vi "led_array.vi"(4 "error in":errorcluster, 7 "LED configuration":string="{\n\t\"actor_id\": \"\",\n\t\"attach_socket\": \"\",\n\t\"description\": \"\",\n\t\"enable_streaming\": true,\n\t\"lights\": [{\n\t\t\"array_id\": \"LF\",\n\t\t\"attach_socket\": \"\",\n\t\t\"coneLights\": [{\n\t\t\t\"attach_socket\": \"\",\n\t\t\t\"attenuation_radius\": 5000.0,\n\t\t\t\"backlight_attenuation_radius\": 20.0,\n\t\t\t\"backlight_color\": {\n\t\t\t\t\"a\": 255,\n\t\t\t\t\"b\": 255,\n\t\t\t\t\"g\": 255,\n\t\t\t\t\"r\": 255\n\t\t\t},\n\t\t\t\"backlight_indirect_lighting_intensity\": 10.0,\n\t\t\t\"backlight_intensity\": 400.0,\n\t\t\t\"backlight_location\": {\n\t\t\t\t\"x\": 0.0,\n\t\t\t\t\"y\": 0.0,\n\t\t\t\t\"z\": 0.0\n\t\t\t},\n\t\t\t\"backlight_soft_source_radius\": 2.0,\n\t\t\t\"backlight_source_length\": 1.0,\n\t\t\t\"backlight_source_radius\": 1.0,\n\t\t\t\"backlight_temperature\": 8000.0,\n\t\t\t\"backlight_volumetric_scattering_intensity\": 10.0,\n\t\t\t\"color\": {\n\t\t\t\t\"a\": 255,\n\t\t\t\t\"b\": 255,\n\t\t\t\t\"g\": 255,\n\t\t\t\t\"r\": 255\n\t\t\t},\n\t\t\t\"description\": \"\",\n\t\t\t\"enable_backlight\": true,\n\t\t\t\"enable_directional_light\": true,\n\t\t\t\"enable_streaming\": true,\n\t\t\t\"ies_profile\": \"\",\n\t\t\t\"indirect_lighting_intensity\": 1.0,\n\t\t\t\"inner_cone_angle\": 2.0,\n\t\t\t\"intensity\": 1500.0,\n\t\t\t\"led\": 0,\n\t\t\t\"listen_port\": 0,\n\t\t\t\"location\": {\n\t\t\t\t\"x\": 0.0,\n\t\t\t\t\"y\": 0.0,\n\t\t\t\t\"z\": 0.0\n\t\t\t},\n\t\t\t\"outer_cone_angle\": 6.0,\n\t\t\t\"parent_component_attachment\": \"\",\n\t\t\t\"raytrace_global_ilum\": false,\n\t\t\t\"raytrace_reflection\": false,\n\t\t\t\"raytrace_shadow\": false,\n\t\t\t\"receive_stream\": true,\n\t\t\t\"rotation\": {\n\t\t\t\t\"pitch\": -1.0,\n\t\t\t\t\"roll\": 0.0,\n\t\t\t\t\"yaw\": 6.0\n\t\t\t},\n\t\t\t\"soft_source_radius\": 0.0,\n\t\t\t\"source_length\": 1.0,\n\t\t\t\"source_radius\": 0.0,\n\t\t\t\"temperature\": 8000.0,\n\t\t\t\"type\": \"None\",\n\t\t\t\"use_attach_socket\": false,\n\t\t\t\"use_parent_component_attachment\": false,\n\t\t\t\"volumetric_scattering_intensity\": 5.0,\n\t\t\t\"wait_for_fresh_frame\": true\n\t\t}, {\n\t\t\t\"attach_socket\": \"\",\n\t\t\t\"attenuation_radius\": 5000.0,\n\t\t\t\"backlight_attenuation_radius\": 20.0,\n\t\t\t\"backlight_color\": {\n\t\t\t\t\"a\": 255,\n\t\t\t\t\"b\": 255,\n\t\t\t\t\"g\": 255,\n\t\t\t\t\"r\": 255\n\t\t\t},\n\t\t\t\"backlight_indirect_lighting_intensity\": 10.0,\n\t\t\t\"backlight_intensity\": 400.0,\n\t\t\t\"backlight_location\": {\n\t\t\t\t\"x\": 0.0,\n\t\t\t\t\"y\": 0.0,\n\t\t\t\t\"z\": 0.0\n\t\t\t},\n\t\t\t\"backlight_soft_source_radius\": 2.0,\n\t\t\t\"backlight_source_length\": 1.0,\n\t\t\t\"backlight_source_radius\": 1.0,\n\t\t\t\"backlight_temperature\": 8000.0,\n\t\t\t\"backlight_volumetric_scattering_intensity\": 10.0,\n\t\t\t\"color\": {\n\t\t\t\t\"a\": 255,\n\t\t\t\t\"b\": 255,\n\t\t\t\t\"g\": 255,\n\t\t\t\t\"r\": 255\n\t\t\t},\n\t\t\t\"description\": \"\",\n\t\t\t\"enable_backlight\": true,\n\t\t\t\"enable_directional_light\": true,\n\t\t\t\"enable_streaming\": true,\n\t\t\t\"ies_profile\": \"\",\n\t\t\t\"indirect_lighting_intensity\": 1.0,\n\t\t\t\"inner_cone_angle\": 2.0,\n\t\t\t\"intensity\": 1500.0,\n\t\t\t\"led\": 1,\n\t\t\t\"listen_port\": 0,\n\t\t\t\"location\": {\n\t\t\t\t\"x\": 0.0,\n\t\t\t\t\"y\": -2.0,\n\t\t\t\t\"z\": 0.0\n\t\t\t},\n\t\t\t\"outer_cone_angle\": 6.0,\n\t\t\t\"parent_component_attachment\": \"\",\n\t\t\t\"raytrace_global_ilum\": false,\n\t\t\t\"raytrace_reflection\": false,\n\t\t\t\"raytrace_shadow\": false,\n\t\t\t\"receive_stream\": true,\n\t\t\t\"rotation\": {\n\t\t\t\t\"pitch\": -1.0,\n\t\t\t\t\"roll\": 0.0,\n\t\t\t\t\"yaw\": 3.0\n\t\t\t},\n\t\t\t\"soft_source_radius\": 0.0,\n\t\t\t\"source_length\": 1.0,\n\t\t\t\"source_radius\": 0.0,\n\t\t\t\"temperature\": 8000.0,\n\t\t\t\"type\": \"None\",\n\t\t\t\"use_attach_socket\": false,\n\t\t\t\"use_parent_component_attachment\": false,\n\t\t\t\"volumetric_scattering_intensity\": 5.0,\n\t\t\t\"wait_for_fresh_frame\": true\n\t\t}, {\n\t\t\t\"attach_socket\": \"\",\n\t\t\t\"attenuation_radius\": 5000.0,\n\t\t\t\"backlight_attenuation_radius\": 20.0,\n\t\t\t\"backlight_color\": {\n\t\t\t\t\"a\": 255,\n\t\t\t\t\"b\": 255,\n\t\t\t\t\"g\": 255,\n\t\t\t\t\"r\": 255\n\t\t\t},\n\t\t\t\"backlight_indirect_lighting_intensity\": 10.0,\n\t\t\t\"backlight_intensity\": 400.0,\n\t\t\t\"backlight_location\": {\n\t\t\t\t\"x\": 0.0,\n\t\t\t\t\"y\": 0.0,\n\t\t\t\t\"z\": 0.0\n\t\t\t},\n\t\t\t\"backlight_soft_source_radius\": 2.0,\n\t\t\t\"backlight_source_length\": 1.0,\n\t\t\t\"backlight_source_radius\": 1.0,\n\t\t\t\"backlight_temperature\": 8000.0,\n\t\t\t\"backlight_volumetric_scattering_intensity\": 10.0,\n\t\t\t\"color\": {\n\t\t\t\t\"a\": 255,\n\t\t\t\t\"b\": 255,\n\t\t\t\t\"g\": 255,\n\t\t\t\t\"r\": 255\n\t\t\t},\n\t\t\t\"description\": \"\",\n\t\t\t\"enable_backlight\": true,\n\t\t\t\"enable_directional_light\": true,\n\t\t\t\"enable_streaming\": true,\n\t\t\t\"ies_profile\": \"\",\n\t\t\t\"indirect_lighting_intensity\": 1.0,\n\t\t\t\"inner_cone_angle\": 2.0,\n\t\t\t\"intensity\": 1500.0,\n\t\t\t\"led\": 2,\n\t\t\t\"listen_port\": 0,\n\t\t\t\"location\": {\n\t\t\t\t\"x\": 0.0,\n\t\t\t\t\"y\": -4.0,\n\t\t\t\t\"z\": 0.0\n\t\t\t},\n\t\t\t\"outer_cone_angle\": 6.0,\n\t\t\t\"parent_component_attachment\": \"\",\n\t\t\t\"raytrace_global_ilum\": false,\n\t\t\t\"raytrace_reflection\": false,\n\t\t\t\"raytrace_shadow\": false,\n\t\t\t\"receive_stream\": true,\n\t\t\t\"rotation\": {\n\t\t\t\t\"pitch\": -1.0,\n\t\t\t\t\"roll\": 0.0,\n\t\t\t\t\"yaw\": 0.0\n\t\t\t},\n\t\t\t\"soft_source_radius\": 0.0,\n\t\t\t\"source_length\": 1.0,\n\t\t\t\"source_radius\": 0.0,\n\t\t\t\"temperature\": 8000.0,\n\t\t\t\"type\": \"None\",\n\t\t\t\"use_attach_socket\": false,\n\t\t\t\"use_parent_component_attachment\": false,\n\t\t\t\"volumetric_scattering_intensity\": 5.0,\n\t\t\t\"wait_for_fresh_frame\": true\n\t\t}, {\n\t\t\t\"attach_socket\": \"\",\n\t\t\t\"attenuation_radius\": 5000.0,\n\t\t\t\"backlight_attenuation_radius\": 20.0,\n\t\t\t\"backlight_color\": {\n\t\t\t\t\"a\": 255,\n\t\t\t\t\"b\": 255,\n\t\t\t\t\"g\": 255,\n\t\t\t\t\"r\": 255\n\t\t\t},\n\t\t\t\"backlight_indirect_lighting_intensity\": 10.0,\n\t\t\t\"backlight_intensity\": 400.0,\n\t\t\t\"backlight_location\": {\n\t\t\t\t\"x\": 0.0,\n\t\t\t\t\"y\": 0.0,\n\t\t\t\t\"z\": 0.0\n\t\t\t},\n\t\t\t\"backlight_soft_source_radius\": 2.0,\n\t\t\t\"backlight_source_length\": 1.0,\n\t\t\t\"backlight_source_radius\": 1.0,\n\t\t\t\"backlight_temperature\": 8000.0,\n\t\t\t\"backlight_volumetric_scattering_intensity\": 10.0,\n\t\t\t\"color\": {\n\t\t\t\t\"a\": 255,\n\t\t\t\t\"b\": 255,\n\t\t\t\t\"g\": 255,\n\t\t\t\t\"r\": 255\n\t\t\t},\n\t\t\t\"description\": \"\",\n\t\t\t\"enable_backlight\": true,\n\t\t\t\"enable_directional_light\": true,\n\t\t\t\"enable_streaming\": true,\n\t\t\t\"ies_profile\": \"\",\n\t\t\t\"indirect_lighting_intensity\": 1.0,\n\t\t\t\"inner_cone_angle\": 2.0,\n\t\t\t\"intensity\": 1500.0,\n\t\t\t\"led\": 3,\n\t\t\t\"listen_port\": 0,\n\t\t\t\"location\": {\n\t\t\t\t\"x\": 0.0,\n\t\t\t\t\"y\": -6.0,\n\t\t\t\t\"z\": 0.0\n\t\t\t},\n\t\t\t\"outer_cone_angle\": 6.0,\n\t\t\t\"parent_component_attachment\": \"\",\n\t\t\t\"raytrace_global_ilum\": false,\n\t\t\t\"raytrace_reflection\": false,\n\t\t\t\"raytrace_shadow\": false,\n\t\t\t\"receive_stream\": true,\n\t\t\t\"rotation\": {\n\t\t\t\t\"pitch\": -1.0,\n\t\t\t\t\"roll\": 0.0,\n\t\t\t\t\"yaw\": -3.0\n\t\t\t},\n\t\t\t\"soft_source_radius\": 0.0,\n\t\t\t\"source_length\": 1.0,\n\t\t\t\"source_radius\": 0.0,\n\t\t\t\"temperature\": 8000.0,\n\t\t\t\"type\": \"None\",\n\t\t\t\"use_attach_socket\": false,\n\t\t\t\"use_parent_component_attachment\": false,\n\t\t\t\"volumetric_scattering_intensity\": 5.0,\n\t\t\t\"wait_for_fresh_frame\": true\n\t\t}, {\n\t\t\t\"attach_socket\": \"\",\n\t\t\t\"attenuation_radius\": 5000.0,\n\t\t\t\"backlight_attenuation_radius\": 20.0,\n\t\t\t\"backlight_color\": {\n\t\t\t\t\"a\": 255,\n\t\t\t\t\"b\": 255,\n\t\t\t\t\"g\": 255,\n\t\t\t\t\"r\": 255\n\t\t\t},\n\t\t\t\"backlight_indirect_lighting_intensity\": 10.0,\n\t\t\t\"backlight_intensity\": 400.0,\n\t\t\t\"backlight_location\": {\n\t\t\t\t\"x\": 0.0,\n\t\t\t\t\"y\": 0.0,\n\t\t\t\t\"z\": 0.0\n\t\t\t},\n\t\t\t\"backlight_soft_source_radius\": 2.0,\n\t\t\t\"backlight_source_length\": 1.0,\n\t\t\t\"backlight_source_radius\": 1.0,\n\t\t\t\"backlight_temperature\": 8000.0,\n\t\t\t\"backlight_volumetric_scattering_intensity\": 10.0,\n\t\t\t\"color\": {\n\t\t\t\t\"a\": 255,\n\t\t\t\t\"b\": 255,\n\t\t\t\t\"g\": 255,\n\t\t\t\t\"r\": 255\n\t\t\t},\n\t\t\t\"description\": \"\",\n\t\t\t\"enable_backlight\": true,\n\t\t\t\"enable_directional_light\": true,\n\t\t\t\"enable_streaming\": true,\n\t\t\t\"ies_profile\": \"\",\n\t\t\t\"indirect_lighting_intensity\": 1.0,\n\t\t\t\"inner_cone_angle\": 2.0,\n\t\t\t\"intensity\": 1500.0,\n\t\t\t\"led\": 4,\n\t\t\t\"listen_port\": 0,\n\t\t\t\"location\": {\n\t\t\t\t\"x\": 0.0,\n\t\t\t\t\"y\": -8.0,\n\t\t\t\t\"z\": 0.0\n\t\t\t},\n\t\t\t\"outer_cone_angle\": 6.0,\n\t\t\t\"parent_component_attachment\": \"\",\n\t\t\t\"raytrace_global_ilum\": false,\n\t\t\t\"raytrace_reflection\": false,\n\t\t\t\"raytrace_shadow\": false,\n\t\t\t\"receive_stream\": true,\n\t\t\t\"rotation\": {\n\t\t\t\t\"pitch\": -1.0,\n\t\t\t\t\"roll\": 0.0,\n\t\t\t\t\"yaw\": -6.0\n\t\t\t},\n\t\t\t\"soft_source_radius\": 0.0,\n\t\t\t\"source_length\": 1.0,\n\t\t\t\"source_radius\": 0.0,\n\t\t\t\"temperature\": 8000.0,\n\t\t\t\"type\": \"None\",\n\t\t\t\"use_attach_socket\": false,\n\t\t\t\"use_parent_component_attachment\": false,\n\t\t\t\"volumetric_scattering_intensity\": 5.0,\n\t\t\t\"wait_for_fresh_frame\": true\n\t\t}, {\n\t\t\t\"attach_socket\": \"\",\n\t\t\t\"attenuation_radius\": 5000.0,\n\t\t\t\"backlight_attenuation_radius\": 20.0,\n\t\t\t\"backlight_color\": {\n\t\t\t\t\"a\": 255,\n\t\t\t\t\"b\": 255,\n\t\t\t\t\"g\": 255,\n\t\t\t\t\"r\": 255\n\t\t\t},\n\t\t\t\"backlight_indirect_lighting_intensity\": 10.0,\n\t\t\t\"backlight_intensity\": 400.0,\n\t\t\t\"backlight_location\": {\n\t\t\t\t\"x\": 0.0,\n\t\t\t\t\"y\": 0.0,\n\t\t\t\t\"z\": 0.0\n\t\t\t},\n\t\t\t\"backlight_soft_source_radius\": 2.0,\n\t\t\t\"backlight_source_length\": 1.0,\n\t\t\t\"backlight_source_radius\": 1.0,\n\t\t\t\"backlight_temperature\": 8000.0,\n\t\t\t\"backlight_volumetric_scattering_intensity\": 10.0,\n\t\t\t\"color\": {\n\t\t\t\t\"a\": 255,\n\t\t\t\t\"b\": 255,\n\t\t\t\t\"g\": 255,\n\t\t\t\t\"r\": 255\n\t\t\t},\n\t\t\t\"description\": \"\",\n\t\t\t\"enable_backlight\": true,\n\t\t\t\"enable_directional_light\": true,\n\t\t\t\"enable_streaming\": true,\n\t\t\t\"ies_profile\": \"\",\n\t\t\t\"indirect_lighting_intensity\": 1.0,\n\t\t\t\"inner_cone_angle\": 2.0,\n\t\t\t\"intensity\": 1500.0,\n\t\t\t\"led\": 5,\n\t\t\t\"listen_port\": 0,\n\t\t\t\"location\": {\n\t\t\t\t\"x\": 0.0,\n\t\t\t\t\"y\": -10.0,\n\t\t\t\t\"z\": 0.0\n\t\t\t},\n\t\t\t\"outer_cone_angle\": 6.0,\n\t\t\t\"parent_component_attachment\": \"\",\n\t\t\t\"raytrace_global_ilum\": false,\n\t\t\t\"raytrace_reflection\": false,\n\t\t\t\"raytrace_shadow\": false,\n\t\t\t\"receive_stream\": true,\n\t\t\t\"rotation\": {\n\t\t\t\t\"pitch\": -1.0,\n\t\t\t\t\"roll\": 0.0,\n\t\t\t\t\"yaw\": -9.0\n\t\t\t},\n\t\t\t\"soft_source_radius\": 0.0,\n\t\t\t\"source_length\": 1.0,\n\t\t\t\"source_radius\": 0.0,\n\t\t\t\"temperature\": 8000.0,\n\t\t\t\"type\": \"None\",\n\t\t\t\"use_attach_socket\": false,\n\t\t\t\"use_parent_component_attachment\": false,\n\t\t\t\"volumetric_scattering_intensity\": 5.0,\n\t\t\t\"wait_for_fresh_frame\": true\n\t\t}, {\n\t\t\t\"attach_socket\": \"\",\n\t\t\t\"attenuation_radius\": 5000.0,\n\t\t\t\"backlight_attenuation_radius\": 20.0,\n\t\t\t\"backlight_color\": {\n\t\t\t\t\"a\": 255,\n\t\t\t\t\"b\": 255,\n\t\t\t\t\"g\": 255,\n\t\t\t\t\"r\": 255\n\t\t\t},\n\t\t\t\"backlight_indirect_lighting_intensity\": 10.0,\n\t\t\t\"backlight_intensity\": 400.0,\n\t\t\t\"backlight_location\": {\n\t\t\t\t\"x\": 0.0,\n\t\t\t\t\"y\": 0.0,\n\t\t\t\t\"z\": 0.0\n\t\t\t},\n\t\t\t\"backlight_soft_source_radius\": 2.0,\n\t\t\t\"backlight_source_length\": 1.0,\n\t\t\t\"backlight_source_radius\": 1.0,\n\t\t\t\"backlight_temperature\": 8000.0,\n\t\t\t\"backlight_volumetric_scattering_intensity\": 10.0,\n\t\t\t\"color\": {\n\t\t\t\t\"a\": 255,\n\t\t\t\t\"b\": 255,\n\t\t\t\t\"g\": 255,\n\t\t\t\t\"r\": 255\n\t\t\t},\n\t\t\t\"description\": \"\",\n\t\t\t\"enable_backlight\": true,\n\t\t\t\"enable_directional_light\": true,\n\t\t\t\"enable_streaming\": true,\n\t\t\t\"ies_profile\": \"\",\n\t\t\t\"indirect_lighting_intensity\": 1.0,\n\t\t\t\"inner_cone_angle\": 2.0,\n\t\t\t\"intensity\": 1500.0,\n\t\t\t\"led\": 6,\n\t\t\t\"listen_port\": 0,\n\t\t\t\"location\": {\n\t\t\t\t\"x\": 0.0,\n\t\t\t\t\"y\": -12.0,\n\t\t\t\t\"z\": 0.0\n\t\t\t},\n\t\t\t\"outer_cone_angle\": 6.0,\n\t\t\t\"parent_component_attachment\": \"\",\n\t\t\t\"raytrace_global_ilum\": false,\n\t\t\t\"raytrace_reflection\": false,\n\t\t\t\"raytrace_shadow\": false,\n\t\t\t\"receive_stream\": true,\n\t\t\t\"rotation\": {\n\t\t\t\t\"pitch\": -1.0,\n\t\t\t\t\"roll\": 0.0,\n\t\t\t\t\"yaw\": -12.0\n\t\t\t},\n\t\t\t\"soft_source_radius\": 0.0,\n\t\t\t\"source_length\": 1.0,\n\t\t\t\"source_radius\": 0.0,\n\t\t\t\"temperature\": 8000.0,\n\t\t\t\"type\": \"None\",\n\t\t\t\"use_attach_socket\": false,\n\t\t\t\"use_parent_component_attachment\": false,\n\t\t\t\"volumetric_scattering_intensity\": 5.0,\n\t\t\t\"wait_for_fresh_frame\": true\n\t\t}, {\n\t\t\t\"attach_socket\": \"\",\n\t\t\t\"attenuation_radius\": 5000.0,\n\t\t\t\"backlight_attenuation_radius\": 20.0,\n\t\t\t\"backlight_color\": {\n\t\t\t\t\"a\": 255,\n\t\t\t\t\"b\": 255,\n\t\t\t\t\"g\": 255,\n\t\t\t\t\"r\": 255\n\t\t\t},\n\t\t\t\"backlight_indirect_lighting_intensity\": 10.0,\n\t\t\t\"backlight_intensity\": 400.0,\n\t\t\t\"backlight_location\": {\n\t\t\t\t\"x\": 0.0,\n\t\t\t\t\"y\": 0.0,\n\t\t\t\t\"z\": 0.0\n\t\t\t},\n\t\t\t\"backlight_soft_source_radius\": 2.0,\n\t\t\t\"backlight_source_length\": 1.0,\n\t\t\t\"backlight_source_radius\": 1.0,\n\t\t\t\"backlight_temperature\": 8000.0,\n\t\t\t\"backlight_volumetric_scattering_intensity\": 10.0,\n\t\t\t\"color\": {\n\t\t\t\t\"a\": 255,\n\t\t\t\t\"b\": 255,\n\t\t\t\t\"g\": 255,\n\t\t\t\t\"r\": 255\n\t\t\t},\n\t\t\t\"description\": \"\",\n\t\t\t\"enable_backlight\": true,\n\t\t\t\"enable_directional_light\": true,\n\t\t\t\"enable_streaming\": true,\n\t\t\t\"ies_profile\": \"\",\n\t\t\t\"indirect_lighting_intensity\": 1.0,\n\t\t\t\"inner_cone_angle\": 2.0,\n\t\t\t\"intensity\": 1500.0,\n\t\t\t\"led\": 7,\n\t\t\t\"listen_port\": 0,\n\t\t\t\"location\": {\n\t\t\t\t\"x\": 0.0,\n\t\t\t\t\"y\": -14.0,\n\t\t\t\t\"z\": 0.0\n\t\t\t},\n\t\t\t\"outer_cone_angle\": 6.0,\n\t\t\t\"parent_component_attachment\": \"\",\n\t\t\t\"raytrace_global_ilum\": false,\n\t\t\t\"raytrace_reflection\": false,\n\t\t\t\"raytrace_shadow\": false,\n\t\t\t\"receive_stream\": true,\n\t\t\t\"rotation\": {\n\t\t\t\t\"pitch\": -1.0,\n\t\t\t\t\"roll\": 0.0,\n\t\t\t\t\"yaw\": -15.0\n\t\t\t},\n\t\t\t\"soft_source_radius\": 0.0,\n\t\t\t\"source_length\": 1.0,\n\t\t\t\"source_radius\": 0.0,\n\t\t\t\"temperature\": 8000.0,\n\t\t\t\"type\": \"None\",\n\t\t\t\"use_attach_socket\": false,\n\t\t\t\"use_parent_component_attachment\": false,\n\t\t\t\"volumetric_scattering_intensity\": 5.0,\n\t\t\t\"wait_for_fresh_frame\": true\n\t\t}],\n\t\t\"description\": \"\",\n\t\t\"enable_streaming\": true,\n\t\t\"listen_port\": 0,\n\t\t\"location\": {\n\t\t\t\"x\": 200.57719399999999155,\n\t\t\t\"y\": -79.397000000000005571,\n\t\t\t\"z\": 83.918998999999999455\n\t\t},\n\t\t\"parent_component_attachment\": \"\",\n\t\t\"receive_stream\": true,\n\t\t\"rectLights\": [],\n\t\t\"rotation\": {\n\t\t\t\"pitch\": 0.0,\n\t\t\t\"roll\": 0.0,\n\t\t\t\"yaw\": 0.0\n\t\t},\n\t\t\"type\": \"None\",\n\t\t\"use_attach_socket\": false,\n\t\t\"use_parent_component_attachment\": false,\n\t\t\"wait_for_fresh_frame\": true\n\t}, {\n\t\t\"array_id\": \"RF\",\n\t\t\"attach_socket\": \"\",\n\t\t\"coneLights\": [{\n\t\t\t\"attach_socket\": \"\",\n\t\t\t\"attenuation_radius\": 5000.0,\n\t\t\t\"backlight_attenuation_radius\": 20.0,\n\t\t\t\"backlight_color\": {\n\t\t\t\t\"a\": 255,\n\t\t\t\t\"b\": 255,\n\t\t\t\t\"g\": 255,\n\t\t\t\t\"r\": 255\n\t\t\t},\n\t\t\t\"backlight_indirect_lighting_intensity\": 10.0,\n\t\t\t\"backlight_intensity\": 400.0,\n\t\t\t\"backlight_location\": {\n\t\t\t\t\"x\": 0.0,\n\t\t\t\t\"y\": 0.0,\n\t\t\t\t\"z\": 0.0\n\t\t\t},\n\t\t\t\"backlight_soft_source_radius\": 2.0,\n\t\t\t\"backlight_source_length\": 1.0,\n\t\t\t\"backlight_source_radius\": 1.0,\n\t\t\t\"backlight_temperature\": 8000.0,\n\t\t\t\"backlight_volumetric_scattering_intensity\": 10.0,\n\t\t\t\"color\": {\n\t\t\t\t\"a\": 255,\n\t\t\t\t\"b\": 255,\n\t\t\t\t\"g\": 255,\n\t\t\t\t\"r\": 255\n\t\t\t},\n\t\t\t\"description\": \"\",\n\t\t\t\"enable_backlight\": true,\n\t\t\t\"enable_directional_light\": true,\n\t\t\t\"enable_streaming\": true,\n\t\t\t\"ies_profile\": \"\",\n\t\t\t\"indirect_lighting_intensity\": 1.0,\n\t\t\t\"inner_cone_angle\": 2.0,\n\t\t\t\"intensity\": 1500.0,\n\t\t\t\"led\": 0,\n\t\t\t\"listen_port\": 0,\n\t\t\t\"location\": {\n\t\t\t\t\"x\": 0.0,\n\t\t\t\t\"y\": 0.0,\n\t\t\t\t\"z\": 0.0\n\t\t\t},\n\t\t\t\"outer_cone_angle\": 6.0,\n\t\t\t\"parent_component_attachment\": \"\",\n\t\t\t\"raytrace_global_ilum\": false,\n\t\t\t\"raytrace_reflection\": false,\n\t\t\t\"raytrace_shadow\": false,\n\t\t\t\"receive_stream\": true,\n\t\t\t\"rotation\": {\n\t\t\t\t\"pitch\": -1.0,\n\t\t\t\t\"roll\": 0.0,\n\t\t\t\t\"yaw\": -6.0\n\t\t\t},\n\t\t\t\"soft_source_radius\": 0.0,\n\t\t\t\"source_length\": 1.0,\n\t\t\t\"source_radius\": 0.0,\n\t\t\t\"temperature\": 8000.0,\n\t\t\t\"type\": \"None\",\n\t\t\t\"use_attach_socket\": false,\n\t\t\t\"use_parent_component_attachment\": false,\n\t\t\t\"volumetric_scattering_intensity\": 5.0,\n\t\t\t\"wait_for_fresh_frame\": true\n\t\t}, {\n\t\t\t\"attach_socket\": \"\",\n\t\t\t\"attenuation_radius\": 5000.0,\n\t\t\t\"backlight_attenuation_radius\": 20.0,\n\t\t\t\"backlight_color\": {\n\t\t\t\t\"a\": 255,\n\t\t\t\t\"b\": 255,\n\t\t\t\t\"g\": 255,\n\t\t\t\t\"r\": 255\n\t\t\t},\n\t\t\t\"backlight_indirect_lighting_intensity\": 10.0,\n\t\t\t\"backlight_intensity\": 400.0,\n\t\t\t\"backlight_location\": {\n\t\t\t\t\"x\": 0.0,\n\t\t\t\t\"y\": 0.0,\n\t\t\t\t\"z\": 0.0\n\t\t\t},\n\t\t\t\"backlight_soft_source_radius\": 2.0,\n\t\t\t\"backlight_source_length\": 1.0,\n\t\t\t\"backlight_source_radius\": 1.0,\n\t\t\t\"backlight_temperature\": 8000.0,\n\t\t\t\"backlight_volumetric_scattering_intensity\": 10.0,\n\t\t\t\"color\": {\n\t\t\t\t\"a\": 255,\n\t\t\t\t\"b\": 255,\n\t\t\t\t\"g\": 255,\n\t\t\t\t\"r\": 255\n\t\t\t},\n\t\t\t\"description\": \"\",\n\t\t\t\"enable_backlight\": true,\n\t\t\t\"enable_directional_light\": true,\n\t\t\t\"enable_streaming\": true,\n\t\t\t\"ies_profile\": \"\",\n\t\t\t\"indirect_lighting_intensity\": 1.0,\n\t\t\t\"inner_cone_angle\": 2.0,\n\t\t\t\"intensity\": 1500.0,\n\t\t\t\"led\": 1,\n\t\t\t\"listen_port\": 0,\n\t\t\t\"location\": {\n\t\t\t\t\"x\": 0.0,\n\t\t\t\t\"y\": 2.0,\n\t\t\t\t\"z\": 0.0\n\t\t\t},\n\t\t\t\"outer_cone_angle\": 6.0,\n\t\t\t\"parent_component_attachment\": \"\",\n\t\t\t\"raytrace_global_ilum\": false,\n\t\t\t\"raytrace_reflection\": false,\n\t\t\t\"raytrace_shadow\": false,\n\t\t\t\"receive_stream\": true,\n\t\t\t\"rotation\": {\n\t\t\t\t\"pitch\": -1.0,\n\t\t\t\t\"roll\": 0.0,\n\t\t\t\t\"yaw\": -3.0\n\t\t\t},\n\t\t\t\"soft_source_radius\": 0.0,\n\t\t\t\"source_length\": 1.0,\n\t\t\t\"source_radius\": 0.0,\n\t\t\t\"temperature\": 8000.0,\n\t\t\t\"type\": \"None\",\n\t\t\t\"use_attach_socket\": false,\n\t\t\t\"use_parent_component_attachment\": false,\n\t\t\t\"volumetric_scattering_intensity\": 5.0,\n\t\t\t\"wait_for_fresh_frame\": true\n\t\t}, {\n\t\t\t\"attach_socket\": \"\",\n\t\t\t\"attenuation_radius\": 5000.0,\n\t\t\t\"backlight_attenuation_radius\": 20.0,\n\t\t\t\"backlight_color\": {\n\t\t\t\t\"a\": 255,\n\t\t\t\t\"b\": 255,\n\t\t\t\t\"g\": 255,\n\t\t\t\t\"r\": 255\n\t\t\t},\n\t\t\t\"backlight_indirect_lighting_intensity\": 10.0,\n\t\t\t\"backlight_intensity\": 400.0,\n\t\t\t\"backlight_location\": {\n\t\t\t\t\"x\": 0.0,\n\t\t\t\t\"y\": 0.0,\n\t\t\t\t\"z\": 0.0\n\t\t\t},\n\t\t\t\"backlight_soft_source_radius\": 2.0,\n\t\t\t\"backlight_source_length\": 1.0,\n\t\t\t\"backlight_source_radius\": 1.0,\n\t\t\t\"backlight_temperature\": 8000.0,\n\t\t\t\"backlight_volumetric_scattering_intensity\": 10.0,\n\t\t\t\"color\": {\n\t\t\t\t\"a\": 255,\n\t\t\t\t\"b\": 255,\n\t\t\t\t\"g\": 255,\n\t\t\t\t\"r\": 255\n\t\t\t},\n\t\t\t\"description\": \"\",\n\t\t\t\"enable_backlight\": true,\n\t\t\t\"enable_directional_light\": true,\n\t\t\t\"enable_streaming\": true,\n\t\t\t\"ies_profile\": \"\",\n\t\t\t\"indirect_lighting_intensity\": 1.0,\n\t\t\t\"inner_cone_angle\": 2.0,\n\t\t\t\"intensity\": 1500.0,\n\t\t\t\"led\": 2,\n\t\t\t\"listen_port\": 0,\n\t\t\t\"location\": {\n\t\t\t\t\"x\": 0.0,\n\t\t\t\t\"y\": 4.0,\n\t\t\t\t\"z\": 0.0\n\t\t\t},\n\t\t\t\"outer_cone_angle\": 6.0,\n\t\t\t\"parent_component_attachment\": \"\",\n\t\t\t\"raytrace_global_ilum\": false,\n\t\t\t\"raytrace_reflection\": false,\n\t\t\t\"raytrace_shadow\": false,\n\t\t\t\"receive_stream\": true,\n\t\t\t\"rotation\": {\n\t\t\t\t\"pitch\": -1.0,\n\t\t\t\t\"roll\": 0.0,\n\t\t\t\t\"yaw\": 0.0\n\t\t\t},\n\t\t\t\"soft_source_radius\": 0.0,\n\t\t\t\"source_length\": 1.0,\n\t\t\t\"source_radius\": 0.0,\n\t\t\t\"temperature\": 8000.0,\n\t\t\t\"type\": \"None\",\n\t\t\t\"use_attach_socket\": false,\n\t\t\t\"use_parent_component_attachment\": false,\n\t\t\t\"volumetric_scattering_intensity\": 5.0,\n\t\t\t\"wait_for_fresh_frame\": true\n\t\t}, {\n\t\t\t\"attach_socket\": \"\",\n\t\t\t\"attenuation_radius\": 5000.0,\n\t\t\t\"backlight_attenuation_radius\": 20.0,\n\t\t\t\"backlight_color\": {\n\t\t\t\t\"a\": 255,\n\t\t\t\t\"b\": 255,\n\t\t\t\t\"g\": 255,\n\t\t\t\t\"r\": 255\n\t\t\t},\n\t\t\t\"backlight_indirect_lighting_intensity\": 10.0,\n\t\t\t\"backlight_intensity\": 400.0,\n\t\t\t\"backlight_location\": {\n\t\t\t\t\"x\": 0.0,\n\t\t\t\t\"y\": 0.0,\n\t\t\t\t\"z\": 0.0\n\t\t\t},\n\t\t\t\"backlight_soft_source_radius\": 2.0,\n\t\t\t\"backlight_source_length\": 1.0,\n\t\t\t\"backlight_source_radius\": 1.0,\n\t\t\t\"backlight_temperature\": 8000.0,\n\t\t\t\"backlight_volumetric_scattering_intensity\": 10.0,\n\t\t\t\"color\": {\n\t\t\t\t\"a\": 255,\n\t\t\t\t\"b\": 255,\n\t\t\t\t\"g\": 255,\n\t\t\t\t\"r\": 255\n\t\t\t},\n\t\t\t\"description\": \"\",\n\t\t\t\"enable_backlight\": true,\n\t\t\t\"enable_directional_light\": true,\n\t\t\t\"enable_streaming\": true,\n\t\t\t\"ies_profile\": \"\",\n\t\t\t\"indirect_lighting_intensity\": 1.0,\n\t\t\t\"inner_cone_angle\": 2.0,\n\t\t\t\"intensity\": 1500.0,\n\t\t\t\"led\": 3,\n\t\t\t\"listen_port\": 0,\n\t\t\t\"location\": {\n\t\t\t\t\"x\": 0.0,\n\t\t\t\t\"y\": 6.0,\n\t\t\t\t\"z\": 0.0\n\t\t\t},\n\t\t\t\"outer_cone_angle\": 6.0,\n\t\t\t\"parent_component_attachment\": \"\",\n\t\t\t\"raytrace_global_ilum\": false,\n\t\t\t\"raytrace_reflection\": false,\n\t\t\t\"raytrace_shadow\": false,\n\t\t\t\"receive_stream\": true,\n\t\t\t\"rotation\": {\n\t\t\t\t\"pitch\": -1.0,\n\t\t\t\t\"roll\": 0.0,\n\t\t\t\t\"yaw\": 3.0\n\t\t\t},\n\t\t\t\"soft_source_radius\": 0.0,\n\t\t\t\"source_length\": 1.0,\n\t\t\t\"source_radius\": 0.0,\n\t\t\t\"temperature\": 8000.0,\n\t\t\t\"type\": \"None\",\n\t\t\t\"use_attach_socket\": false,\n\t\t\t\"use_parent_component_attachment\": false,\n\t\t\t\"volumetric_scattering_intensity\": 5.0,\n\t\t\t\"wait_for_fresh_frame\": true\n\t\t}, {\n\t\t\t\"attach_socket\": \"\",\n\t\t\t\"attenuation_radius\": 5000.0,\n\t\t\t\"backlight_attenuation_radius\": 20.0,\n\t\t\t\"backlight_color\": {\n\t\t\t\t\"a\": 255,\n\t\t\t\t\"b\": 255,\n\t\t\t\t\"g\": 255,\n\t\t\t\t\"r\": 255\n\t\t\t},\n\t\t\t\"backlight_indirect_lighting_intensity\": 10.0,\n\t\t\t\"backlight_intensity\": 400.0,\n\t\t\t\"backlight_location\": {\n\t\t\t\t\"x\": 0.0,\n\t\t\t\t\"y\": 0.0,\n\t\t\t\t\"z\": 0.0\n\t\t\t},\n\t\t\t\"backlight_soft_source_radius\": 2.0,\n\t\t\t\"backlight_source_length\": 1.0,\n\t\t\t\"backlight_source_radius\": 1.0,\n\t\t\t\"backlight_temperature\": 8000.0,\n\t\t\t\"backlight_volumetric_scattering_intensity\": 10.0,\n\t\t\t\"color\": {\n\t\t\t\t\"a\": 255,\n\t\t\t\t\"b\": 255,\n\t\t\t\t\"g\": 255,\n\t\t\t\t\"r\": 255\n\t\t\t},\n\t\t\t\"description\": \"\",\n\t\t\t\"enable_backlight\": true,\n\t\t\t\"enable_directional_light\": true,\n\t\t\t\"enable_streaming\": true,\n\t\t\t\"ies_profile\": \"\",\n\t\t\t\"indirect_lighting_intensity\": 1.0,\n\t\t\t\"inner_cone_angle\": 2.0,\n\t\t\t\"intensity\": 1500.0,\n\t\t\t\"led\": 4,\n\t\t\t\"listen_port\": 0,\n\t\t\t\"location\": {\n\t\t\t\t\"x\": 0.0,\n\t\t\t\t\"y\": 8.0,\n\t\t\t\t\"z\": 0.0\n\t\t\t},\n\t\t\t\"outer_cone_angle\": 6.0,\n\t\t\t\"parent_component_attachment\": \"\",\n\t\t\t\"raytrace_global_ilum\": false,\n\t\t\t\"raytrace_reflection\": false,\n\t\t\t\"raytrace_shadow\": false,\n\t\t\t\"receive_stream\": true,\n\t\t\t\"rotation\": {\n\t\t\t\t\"pitch\": -1.0,\n\t\t\t\t\"roll\": 0.0,\n\t\t\t\t\"yaw\": 6.0\n\t\t\t},\n\t\t\t\"soft_source_radius\": 0.0,\n\t\t\t\"source_length\": 1.0,\n\t\t\t\"source_radius\": 0.0,\n\t\t\t\"temperature\": 8000.0,\n\t\t\t\"type\": \"None\",\n\t\t\t\"use_attach_socket\": false,\n\t\t\t\"use_parent_component_attachment\": false,\n\t\t\t\"volumetric_scattering_intensity\": 5.0,\n\t\t\t\"wait_for_fresh_frame\": true\n\t\t}, {\n\t\t\t\"attach_socket\": \"\",\n\t\t\t\"attenuation_radius\": 5000.0,\n\t\t\t\"backlight_attenuation_radius\": 20.0,\n\t\t\t\"backlight_color\": {\n\t\t\t\t\"a\": 255,\n\t\t\t\t\"b\": 255,\n\t\t\t\t\"g\": 255,\n\t\t\t\t\"r\": 255\n\t\t\t},\n\t\t\t\"backlight_indirect_lighting_intensity\": 10.0,\n\t\t\t\"backlight_intensity\": 400.0,\n\t\t\t\"backlight_location\": {\n\t\t\t\t\"x\": 0.0,\n\t\t\t\t\"y\": 0.0,\n\t\t\t\t\"z\": 0.0\n\t\t\t},\n\t\t\t\"backlight_soft_source_radius\": 2.0,\n\t\t\t\"backlight_source_length\": 1.0,\n\t\t\t\"backlight_source_radius\": 1.0,\n\t\t\t\"backlight_temperature\": 8000.0,\n\t\t\t\"backlight_volumetric_scattering_intensity\": 10.0,\n\t\t\t\"color\": {\n\t\t\t\t\"a\": 255,\n\t\t\t\t\"b\": 255,\n\t\t\t\t\"g\": 255,\n\t\t\t\t\"r\": 255\n\t\t\t},\n\t\t\t\"description\": \"\",\n\t\t\t\"enable_backlight\": true,\n\t\t\t\"enable_directional_light\": true,\n\t\t\t\"enable_streaming\": true,\n\t\t\t\"ies_profile\": \"\",\n\t\t\t\"indirect_lighting_intensity\": 1.0,\n\t\t\t\"inner_cone_angle\": 2.0,\n\t\t\t\"intensity\": 1500.0,\n\t\t\t\"led\": 5,\n\t\t\t\"listen_port\": 0,\n\t\t\t\"location\": {\n\t\t\t\t\"x\": 0.0,\n\t\t\t\t\"y\": 10.0,\n\t\t\t\t\"z\": 0.0\n\t\t\t},\n\t\t\t\"outer_cone_angle\": 6.0,\n\t\t\t\"parent_component_attachment\": \"\",\n\t\t\t\"raytrace_global_ilum\": false,\n\t\t\t\"raytrace_reflection\": false,\n\t\t\t\"raytrace_shadow\": false,\n\t\t\t\"receive_stream\": true,\n\t\t\t\"rotation\": {\n\t\t\t\t\"pitch\": -1.0,\n\t\t\t\t\"roll\": 0.0,\n\t\t\t\t\"yaw\": 9.0\n\t\t\t},\n\t\t\t\"soft_source_radius\": 0.0,\n\t\t\t\"source_length\": 1.0,\n\t\t\t\"source_radius\": 0.0,\n\t\t\t\"temperature\": 8000.0,\n\t\t\t\"type\": \"None\",\n\t\t\t\"use_attach_socket\": false,\n\t\t\t\"use_parent_component_attachment\": false,\n\t\t\t\"volumetric_scattering_intensity\": 5.0,\n\t\t\t\"wait_for_fresh_frame\": true\n\t\t}, {\n\t\t\t\"attach_socket\": \"\",\n\t\t\t\"attenuation_radius\": 5000.0,\n\t\t\t\"backlight_attenuation_radius\": 20.0,\n\t\t\t\"backlight_color\": {\n\t\t\t\t\"a\": 255,\n\t\t\t\t\"b\": 255,\n\t\t\t\t\"g\": 255,\n\t\t\t\t\"r\": 255\n\t\t\t},\n\t\t\t\"backlight_indirect_lighting_intensity\": 10.0,\n\t\t\t\"backlight_intensity\": 400.0,\n\t\t\t\"backlight_location\": {\n\t\t\t\t\"x\": 0.0,\n\t\t\t\t\"y\": 0.0,\n\t\t\t\t\"z\": 0.0\n\t\t\t},\n\t\t\t\"backlight_soft_source_radius\": 2.0,\n\t\t\t\"backlight_source_length\": 1.0,\n\t\t\t\"backlight_source_radius\": 1.0,\n\t\t\t\"backlight_temperature\": 8000.0,\n\t\t\t\"backlight_volumetric_scattering_intensity\": 10.0,\n\t\t\t\"color\": {\n\t\t\t\t\"a\": 255,\n\t\t\t\t\"b\": 255,\n\t\t\t\t\"g\": 255,\n\t\t\t\t\"r\": 255\n\t\t\t},\n\t\t\t\"description\": \"\",\n\t\t\t\"enable_backlight\": true,\n\t\t\t\"enable_directional_light\": true,\n\t\t\t\"enable_streaming\": true,\n\t\t\t\"ies_profile\": \"\",\n\t\t\t\"indirect_lighting_intensity\": 1.0,\n\t\t\t\"inner_cone_angle\": 2.0,\n\t\t\t\"intensity\": 1500.0,\n\t\t\t\"led\": 6,\n\t\t\t\"listen_port\": 0,\n\t\t\t\"location\": {\n\t\t\t\t\"x\": 0.0,\n\t\t\t\t\"y\": 12.0,\n\t\t\t\t\"z\": 0.0\n\t\t\t},\n\t\t\t\"outer_cone_angle\": 6.0,\n\t\t\t\"parent_component_attachment\": \"\",\n\t\t\t\"raytrace_global_ilum\": false,\n\t\t\t\"raytrace_reflection\": false,\n\t\t\t\"raytrace_shadow\": false,\n\t\t\t\"receive_stream\": true,\n\t\t\t\"rotation\": {\n\t\t\t\t\"pitch\": -1.0,\n\t\t\t\t\"roll\": 0.0,\n\t\t\t\t\"yaw\": 12.0\n\t\t\t},\n\t\t\t\"soft_source_radius\": 0.0,\n\t\t\t\"source_length\": 1.0,\n\t\t\t\"source_radius\": 0.0,\n\t\t\t\"temperature\": 8000.0,\n\t\t\t\"type\": \"None\",\n\t\t\t\"use_attach_socket\": false,\n\t\t\t\"use_parent_component_attachment\": false,\n\t\t\t\"volumetric_scattering_intensity\": 5.0,\n\t\t\t\"wait_for_fresh_frame\": true\n\t\t}, {\n\t\t\t\"attach_socket\": \"\",\n\t\t\t\"attenuation_radius\": 5000.0,\n\t\t\t\"backlight_attenuation_radius\": 20.0,\n\t\t\t\"backlight_color\": {\n\t\t\t\t\"a\": 255,\n\t\t\t\t\"b\": 255,\n\t\t\t\t\"g\": 255,\n\t\t\t\t\"r\": 255\n\t\t\t},\n\t\t\t\"backlight_indirect_lighting_intensity\": 10.0,\n\t\t\t\"backlight_intensity\": 400.0,\n\t\t\t\"backlight_location\": {\n\t\t\t\t\"x\": 0.0,\n\t\t\t\t\"y\": 0.0,\n\t\t\t\t\"z\": 0.0\n\t\t\t},\n\t\t\t\"backlight_soft_source_radius\": 2.0,\n\t\t\t\"backlight_source_length\": 1.0,\n\t\t\t\"backlight_source_radius\": 1.0,\n\t\t\t\"backlight_temperature\": 8000.0,\n\t\t\t\"backlight_volumetric_scattering_intensity\": 10.0,\n\t\t\t\"color\": {\n\t\t\t\t\"a\": 255,\n\t\t\t\t\"b\": 255,\n\t\t\t\t\"g\": 255,\n\t\t\t\t\"r\": 255\n\t\t\t},\n\t\t\t\"description\": \"\",\n\t\t\t\"enable_backlight\": true,\n\t\t\t\"enable_directional_light\": true,\n\t\t\t\"enable_streaming\": true,\n\t\t\t\"ies_profile\": \"\",\n\t\t\t\"indirect_lighting_intensity\": 1.0,\n\t\t\t\"inner_cone_angle\": 2.0,\n\t\t\t\"intensity\": 1500.0,\n\t\t\t\"led\": 7,\n\t\t\t\"listen_port\": 0,\n\t\t\t\"location\": {\n\t\t\t\t\"x\": 0.0,\n\t\t\t\t\"y\": 14.0,\n\t\t\t\t\"z\": 0.0\n\t\t\t},\n\t\t\t\"outer_cone_angle\": 6.0,\n\t\t\t\"parent_component_attachment\": \"\",\n\t\t\t\"raytrace_global_ilum\": false,\n\t\t\t\"raytrace_reflection\": false,\n\t\t\t\"raytrace_shadow\": false,\n\t\t\t\"receive_stream\": true,\n\t\t\t\"rotation\": {\n\t\t\t\t\"pitch\": -1.0,\n\t\t\t\t\"roll\": 0.0,\n\t\t\t\t\"yaw\": 15.0\n\t\t\t},\n\t\t\t\"soft_source_radius\": 0.0,\n\t\t\t\"source_length\": 1.0,\n\t\t\t\"source_radius\": 0.0,\n\t\t\t\"temperature\": 8000.0,\n\t\t\t\"type\": \"None\",\n\t\t\t\"use_attach_socket\": false,\n\t\t\t\"use_parent_component_attachment\": false,\n\t\t\t\"volumetric_scattering_intensity\": 5.0,\n\t\t\t\"wait_for_fresh_frame\": true\n\t\t}],\n\t\t\"description\": \"\",\n\t\t\"enable_streaming\": true,\n\t\t\"listen_port\": 0,\n\t\t\"location\": {\n\t\t\t\"x\": 200.57719399999999155,\n\t\t\t\"y\": 79.397000000000005571,\n\t\t\t\"z\": 83.918998999999999455\n\t\t},\n\t\t\"parent_component_attachment\": \"\",\n\t\t\"receive_stream\": true,\n\t\t\"rectLights\": [],\n\t\t\"rotation\": {\n\t\t\t\"pitch\": 0.0,\n\t\t\t\"roll\": 0.0,\n\t\t\t\"yaw\": 0.0\n\t\t},\n\t\t\"type\": \"None\",\n\t\t\"use_attach_socket\": false,\n\t\t\"use_parent_component_attachment\": false,\n\t\t\"wait_for_fresh_frame\": true\n\t}],\n\t\"listen_port\": 0,\n\t\"location\": {\n\t\t\"x\": 0.0,\n\t\t\"y\": 0.0,\n\t\t\"z\": 0.0\n\t},\n\t\"parent_component_attachment\": \"\",\n\t\"receive_stream\": true,\n\t\"rotation\": {\n\t\t\"pitch\": 0.0,\n\t\t\"roll\": 0.0,\n\t\t\"yaw\": 0.0\n\t},\n\t\"type\": \"None\",\n\t\"use_attach_socket\": false,\n\t\"use_parent_component_attachment\": false,\n\t\"wait_for_fresh_frame\": true\n}") -> (0 "error out":errorcluster)   [LabVIEW 2019]
doc: "Configures and updates an array of LEDs attached to the ego vehicle."
uses:
  controls/lights_state.ctl
  controls/lights_rect_cone.ctl
  tools/simx_common.vi
panel:
  out "Number of Lights Detected":i32=16
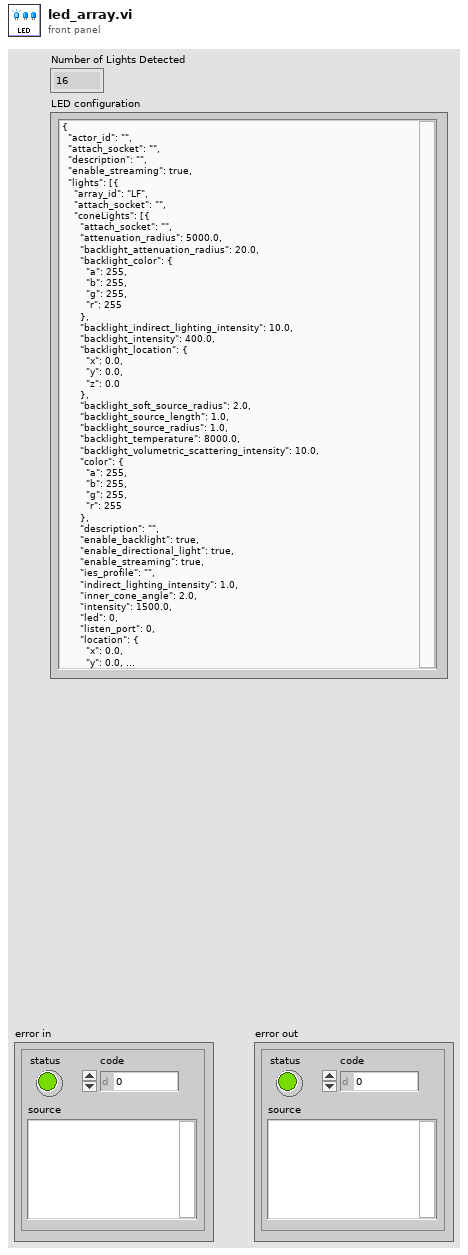
[diagram p1: front panel]
types:
  T1 = typedef "lights_state.ctl" = enum16{"Init", "Configure", "Update"}
  T2 = typedef "simx_connection.ctl" = cluster{"Config":T3, "Connections":T6, "Map":cluster{"lanes":cluster{"x":dbl[], "y":dbl[], "z":dbl[]}, "StartPosition":cluster{"start_points":T7, "StartRotation":dbl[], "StartLocation":dbl[]}, "Draw Map Size":T8, "DrawArea":cluster{"min_Y":dbl, "min_X":dbl, "Scale X":dbl, "Scale Y":dbl}, "Map":picture, "Map Geojson":string}}
  T3 = typedef "config.ctl" = cluster{"Trajectory":T4, "Weather":T5}
  T4 = typedef "trajectory.ctl" = cluster{"Number of frames":i32, "Frame number":i32, "Trajectory":string}
  T5 = typedef "weather.ctl" = cluster{"id":string}
  T6 = typedef "connections.ctl" = cluster{"Simulator Connection":refnum<k5>, "server_ip":string, "Port":i32, "Sensor connections":refnum<k5>[]}
  T7 = typedef "start_points.ctl" = cluster{"locations":dbl[][], "rotations":dbl[][], "type":string[]}
  T8 = typedef "LVBoundsTypeDef.ctl" = cluster{"Width":u32, "Height":u32}
  T9 = cluster{"actor_id":string, "lights":cluster{"array_id":string, "coneLights":cluster{"backlight_intensity":sgl, "intensity":sgl, "led":i32}[]}[]}
  T10 = typedef "lights_rect_cone.ctl" = cluster{"actor_id":string, "lights":cluster{"array_id":string, "coneLights":cluster{"attach_socket":string, "attenuation_radius":sgl, "backlight_attenuation_radius":sgl, "backlight_color":cluster{"a":i32, "b":i32, "g":i32, "r":i32}, "backlight_indirect_lighting_intensity":sgl, "backlight_intensity":sgl, "backlight_location":cluster{"x":sgl, "y":sgl, "z":sgl}, "backlight_soft_source_radius":sgl, "backlight_source_length":sgl, "backlight_source_radius":sgl, "backlight_temperature":sgl, "backlight_volumetric_scattering_intensity":sgl, "color":cluster{"a":i32, "b":i32, "g":i32, "r":i32}, "description":string, "enable_backlight":bool, "enable_directional_light":bool, "enable_streaming":bool, "ies_profile":string, "indirect_lighting_intensity":sgl, "inner_cone_angle":sgl, "intensity":sgl, "led":i32, "listen_port":i32, "location":cluster{"x":sgl, "y":sgl, "z":sgl}, "outer_cone_angle":sgl, "parent_component_attachment":string, "raytrace_global_ilum":bool, "raytrace_reflection":bool, "raytrace_shadow":bool, "receive_stream":bool, "rotation":cluster{"pitch":sgl, "roll":sgl, "yaw":sgl}, "soft_source_radius":sgl, "source_length":sgl, "source_radius":sgl, "temperature":sgl, "type":string, "use_attach_socket":bool, "use_parent_component_attachment":bool, "volumetric_scattering_intensity":sgl, "wait_for_fresh_frame":bool}[], "location":cluster{"x":sgl, "y":sgl, "z":sgl}, "rectLights":cluster{"attach_socket":string, "attenuation_radius":sgl, "backlight_attenuation_radius":sgl, "backlight_color":cluster{"a":i32, "b":i32, "g":i32, "r":i32}, "backlight_indirect_lighting_intensity":sgl, "backlight_intensity":sgl, "backlight_location":cluster{"x":sgl, "y":sgl, "z":sgl}, "backlight_soft_source_radius":sgl, "backlight_source_length":sgl, "backlight_source_radius":sgl, "backlight_temperature":sgl, "backlight_volumetric_scattering_intensity":sgl, "color":cluster{"a":i32, "b":i32, "g":i32, "r":i32}, "description":string, "enable_backlight":bool, "enable_directional_light":bool, "enable_streaming":bool, "ies_profile":string, "indirect_lighting_intensity":sgl, "intensity":sgl, "led":i32, "listen_port":i32, "location":cluster{"x":sgl, "y":sgl, "z":sgl}, "parent_component_attachment":string, "raytrace_global_ilum":bool, "raytrace_reflection":bool, "raytrace_shadow":bool, "receive_stream":bool, "rotation":cluster{"pitch":sgl, "roll":sgl, "yaw":sgl}, "source_height":sgl, "source_width":sgl, "temperature":sgl, "type":string, "use_attach_socket":bool, "use_parent_component_attachment":bool, "volumetric_scattering_intensity":sgl, "wait_for_fresh_frame":bool}[], "rotation":cluster{"pitch":i32, "roll":i32, "yaw":i32}}[]}
  T11 = cluster{"array_id":string, "coneLights":cluster{"backlight_intensity":sgl, "intensity":sgl, "led":i32}[]}
  T12 = cluster{"array_id":string, "coneLights":cluster{"backlight_intensity":sgl, "intensity":sgl, "led":i32}[]}[]
  T13 = cluster{"backlight_intensity":sgl, "intensity":sgl, "led":i32}[]
  T14 = cluster{"backlight_intensity":sgl, "intensity":sgl, "led":i32}
  T15 = cluster{"array_id":string, "coneLights":cluster{"attach_socket":string, "attenuation_radius":sgl, "backlight_attenuation_radius":sgl, "backlight_color":cluster{"a":i32, "b":i32, "g":i32, "r":i32}, "backlight_indirect_lighting_intensity":sgl, "backlight_intensity":sgl, "backlight_location":cluster{"x":sgl, "y":sgl, "z":sgl}, "backlight_soft_source_radius":sgl, "backlight_source_length":sgl, "backlight_source_radius":sgl, "backlight_temperature":sgl, "backlight_volumetric_scattering_intensity":sgl, "color":cluster{"a":i32, "b":i32, "g":i32, "r":i32}, "description":string, "enable_backlight":bool, "enable_directional_light":bool, "enable_streaming":bool, "ies_profile":string, "indirect_lighting_intensity":sgl, "inner_cone_angle":sgl, "intensity":sgl, "led":i32, "listen_port":i32, "location":cluster{"x":sgl, "y":sgl, "z":sgl}, "outer_cone_angle":sgl, "parent_component_attachment":string, "raytrace_global_ilum":bool, "raytrace_reflection":bool, "raytrace_shadow":bool, "receive_stream":bool, "rotation":cluster{"pitch":sgl, "roll":sgl, "yaw":sgl}, "soft_source_radius":sgl, "source_length":sgl, "source_radius":sgl, "temperature":sgl, "type":string, "use_attach_socket":bool, "use_parent_component_attachment":bool, "volumetric_scattering_intensity":sgl, "wait_for_fresh_frame":bool}[], "location":cluster{"x":sgl, "y":sgl, "z":sgl}, "rectLights":cluster{"attach_socket":string, "attenuation_radius":sgl, "backlight_attenuation_radius":sgl, "backlight_color":cluster{"a":i32, "b":i32, "g":i32, "r":i32}, "backlight_indirect_lighting_intensity":sgl, "backlight_intensity":sgl, "backlight_location":cluster{"x":sgl, "y":sgl, "z":sgl}, "backlight_soft_source_radius":sgl, "backlight_source_length":sgl, "backlight_source_radius":sgl, "backlight_temperature":sgl, "backlight_volumetric_scattering_intensity":sgl, "color":cluster{"a":i32, "b":i32, "g":i32, "r":i32}, "description":string, "enable_backlight":bool, "enable_directional_light":bool, "enable_streaming":bool, "ies_profile":string, "indirect_lighting_intensity":sgl, "intensity":sgl, "led":i32, "listen_port":i32, "location":cluster{"x":sgl, "y":sgl, "z":sgl}, "parent_component_attachment":string, "raytrace_global_ilum":bool, "raytrace_reflection":bool, "raytrace_shadow":bool, "receive_stream":bool, "rotation":cluster{"pitch":sgl, "roll":sgl, "yaw":sgl}, "source_height":sgl, "source_width":sgl, "temperature":sgl, "type":string, "use_attach_socket":bool, "use_parent_component_attachment":bool, "volumetric_scattering_intensity":sgl, "wait_for_fresh_frame":bool}[], "rotation":cluster{"pitch":i32, "roll":i32, "yaw":i32}}[]
  T16 = cluster{"attach_socket":string, "attenuation_radius":sgl, "backlight_attenuation_radius":sgl, "backlight_color":cluster{"a":i32, "b":i32, "g":i32, "r":i32}, "backlight_indirect_lighting_intensity":sgl, "backlight_intensity":sgl, "backlight_location":cluster{"x":sgl, "y":sgl, "z":sgl}, "backlight_soft_source_radius":sgl, "backlight_source_length":sgl, "backlight_source_radius":sgl, "backlight_temperature":sgl, "backlight_volumetric_scattering_intensity":sgl, "color":cluster{"a":i32, "b":i32, "g":i32, "r":i32}, "description":string, "enable_backlight":bool, "enable_directional_light":bool, "enable_streaming":bool, "ies_profile":string, "indirect_lighting_intensity":sgl, "inner_cone_angle":sgl, "intensity":sgl, "led":i32, "listen_port":i32, "location":cluster{"x":sgl, "y":sgl, "z":sgl}, "outer_cone_angle":sgl, "parent_component_attachment":string, "raytrace_global_ilum":bool, "raytrace_reflection":bool, "raytrace_shadow":bool, "receive_stream":bool, "rotation":cluster{"pitch":sgl, "roll":sgl, "yaw":sgl}, "soft_source_radius":sgl, "source_length":sgl, "source_radius":sgl, "temperature":sgl, "type":string, "use_attach_socket":bool, "use_parent_component_attachment":bool, "volumetric_scattering_intensity":sgl, "wait_for_fresh_frame":bool}[]
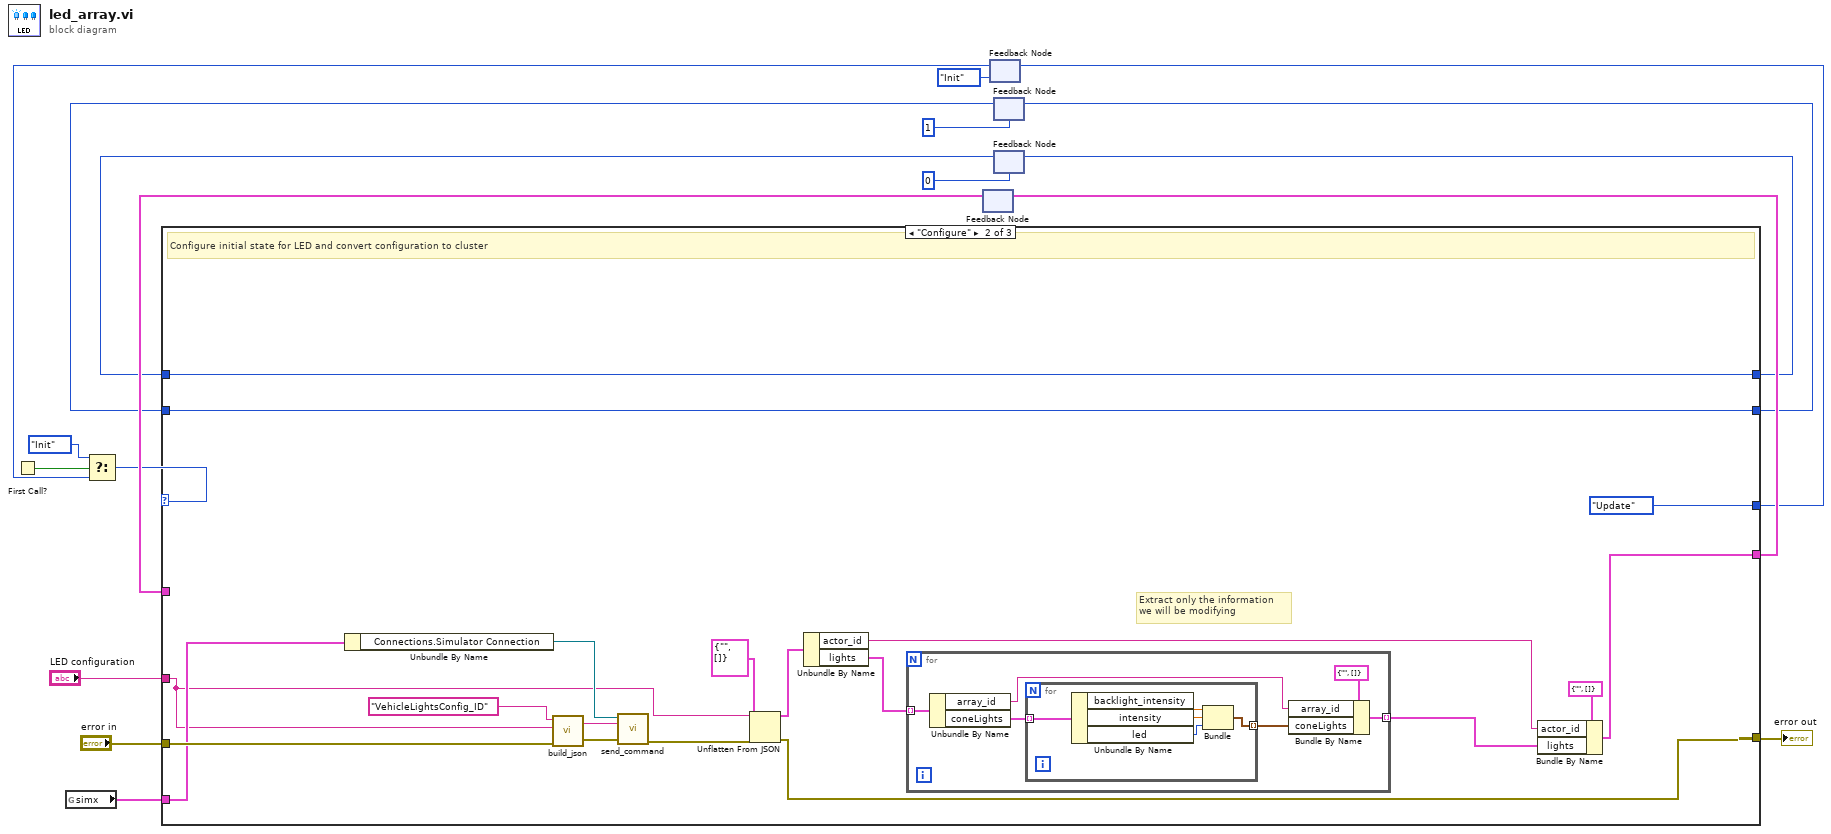
[diagram p0: block diagram]
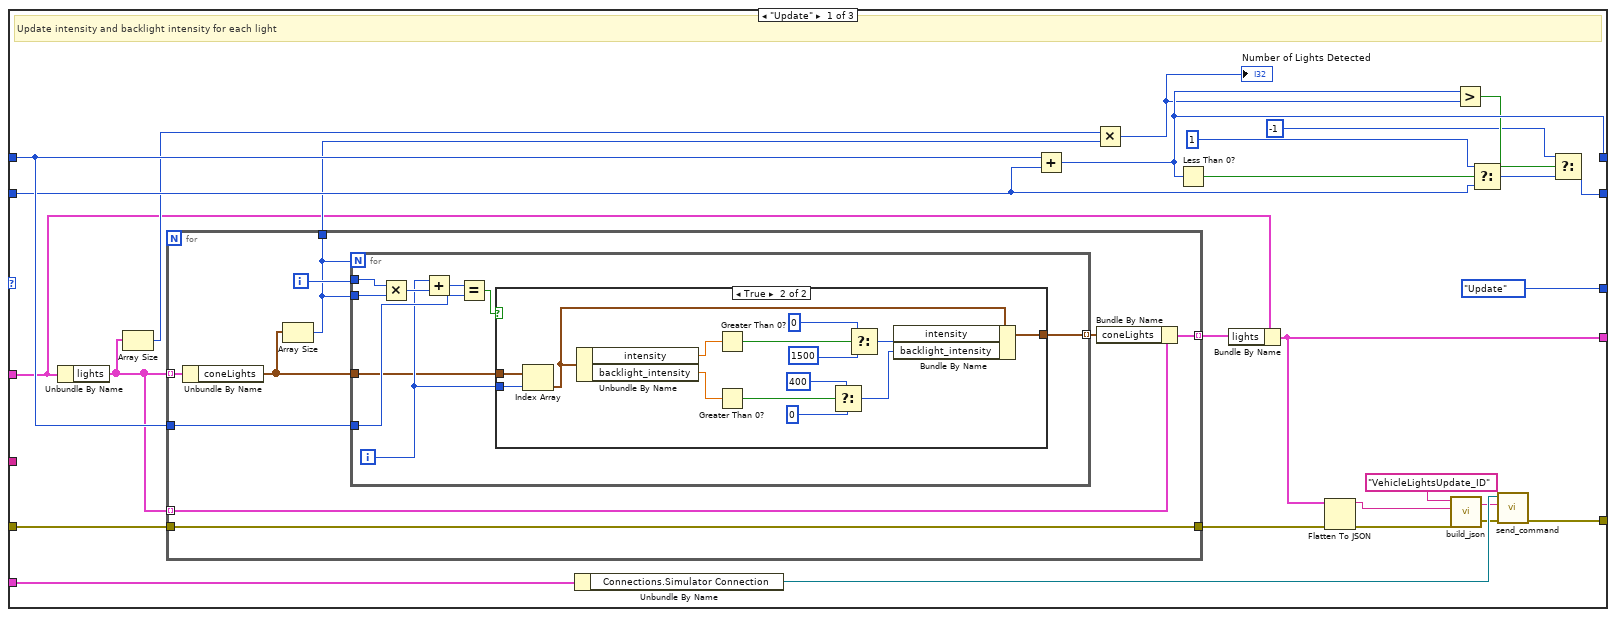
[diagram p2: hidden frame]
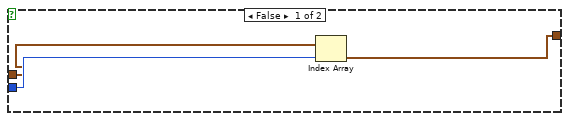
[diagram p3: hidden frame]
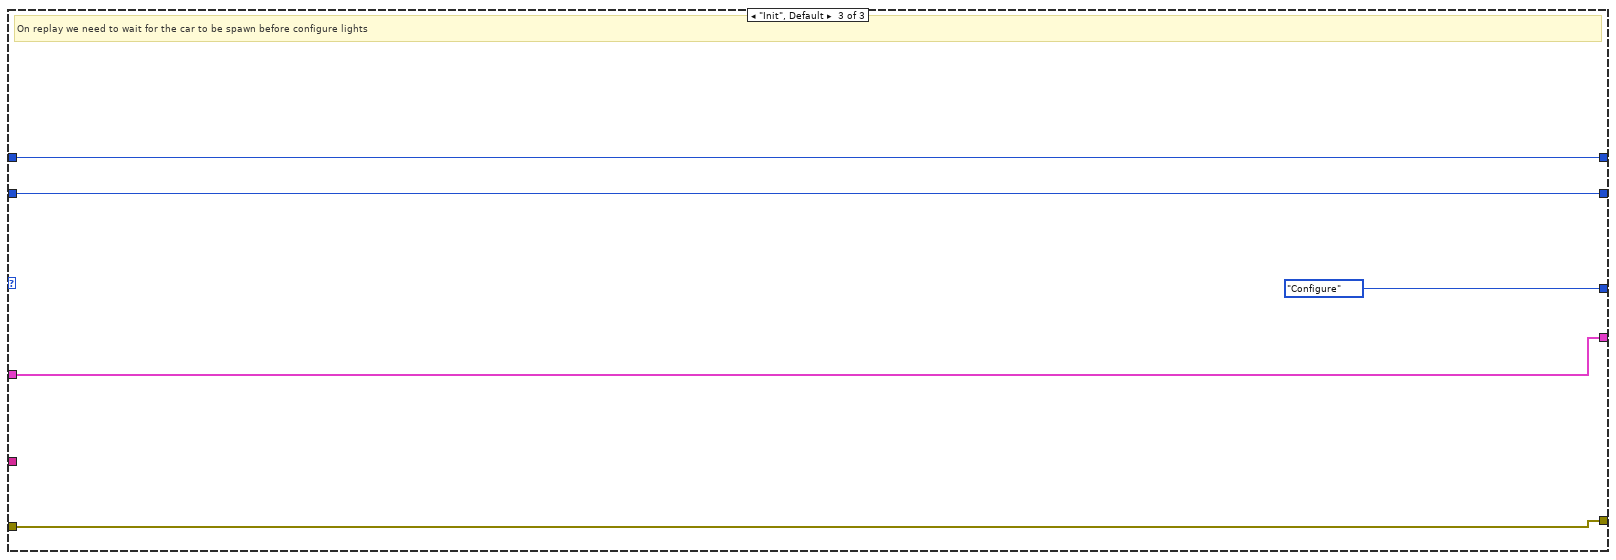
[diagram p4: hidden frame]
diagram:
  n1 = First Call?() -> (First Call?: T/F=w4:bool)
  n2 = global read "simx_common.vi" "simx"() -> (w13:T2)
  n3 = feedback #1() -> (w12:T9)  [unwired: 1 in]
  n4 = feedback #2(lights_state."Init") -> (w2:T1)
  n5 = Select(t=lights_state."Init", s=w4, f=w2) -> (s? t:f=w5:T1)
  n6 = feedback #3(1 ("delta")) -> (w7:i32)
  n7 = feedback #4(0 ("led_index")) -> (w10:i32)
  n8 = case shown="\"Configure\"" w5 {
    tunnel: "LED configuration" -> [_ w88 _]
    tunnel: "error in" -> [w43 w99 w111]
    tunnel: w13 -> [w45 w98 _]
    tunnel: [w44 w97 w111] -> w18
    tunnel: w12 -> [w21 _ w114]
    tunnel: [w20 w81 w114] -> w11
    tunnel: w7 -> [w39 w91 w113]
    tunnel: w10 -> [w40 w90 w112]
    tunnel: [w42 w90 w112] -> w9
    tunnel: [w41 w91 w113] -> w8
    tunnel: [lights_state."Update" lights_state."Update" lights_state."Configure"] -> w3
    frame "Update" {
      # "Update intensity and backlight intensity for each light"
      n9 = Unbundle By Name(w21) -> ("lights"=w19:T12)
      n10 = Array Size(array=w19) -> (size(s)=w25:i32)
      n11 = for {
        tunnel: [w51] -> w22 mode=indexing
        tunnel: w40 -> [w53]
        tunnel: w43 -> [w50]
        tunnel: [w50] -> w37
        tunnel: [w49] -> w24
        tunnel: w19 -> [w48] mode=indexing
        tunnel: w19 -> [w47] mode=indexing
        i -> [w52]
        n12 = Unbundle By Name(w48) -> ("coneLights"=w46:T13)
        n13 = Array Size(array=w46) -> (size(s)=w49:i32)
        n14 = for {
          N: w49 -> [_]
          tunnel: [w63] -> w54 mode=indexing
          tunnel: w52 -> [w62]
          tunnel: w53 -> [w60]
          tunnel: w49 -> [w58]
          tunnel: w46 -> [w55]
          i -> [w56]
          n15 = Multiply(x=w62, y=w58) -> (x*y=w61:i32)
          n16 = Add(x=w56, y=w61) -> (x+y=w57:i32)
          n17 = Equal?(x=w57, y=w60) -> (x = y?=w59:bool)
          n18 = case shown="True" w59 {
            tunnel: [w65 w80] -> w63
            tunnel: w56 -> [w66 w73]
            tunnel: w55 -> [w64 w70]
            frame False {
              n19 = Index Array(array=w64, index=w66) -> (element=w65:T14)
            }
            frame True {
              n20 = Index Array(array=w70, index=w73) -> (element=w67:T14)
              n21 = Unbundle By Name(w67) -> ("intensity"=w69:sgl, "backlight_intensity"=w68:sgl)
              n22 = Greater Than 0?(x=w69) -> (x > 0?=w77:bool)
              n23 = Greater Than 0?(x=w68) -> (x > 0?=w75:bool)
              n24 = Select(t=400 ("intensity"), s=w75, f=0) -> (s? t:f=w74:i32)
              n25 = Select(t=0 ("intensity"), s=w77, f=1500) -> (s? t:f=w72:i32)
              n26 = Bundle By Name(cluster=w67, "intensity"=w72, "backlight_intensity"=w74) -> (w80:T14)
            }
          }
        }
        n27 = Bundle By Name(cluster=w47, "coneLights"=w54) -> (w51:T11)
      }
      n28 = Unbundle By Name(w45) -> ("Connections.Simulator Connection"=w38:refnum<k5>)
      n29 = Add(x=w40, y=w39) -> (x+y=w42:i32)
      n30 = Multiply(x=w25, y=w24) -> (x*y=w23:i32)
      "Number of Lights Detected" <- w23
      n31 = Less Than 0?(x=w42) -> (x < 0?=w30:bool)
      n32 = Bundle By Name(cluster=w21, "lights"=w22) -> (w20:T9)
      n33 = Flatten To JSON(anything=w20, error in (no error)=w37) -> (JSON string=w35:string, 11:w36:errorcluster)  [unwired: 1 in]
      n34 = call "build_json.vi"("error in"=w36, "Message"=w35, "Command_ID"="VehicleLightsUpdate_ID") -> ("error out"=w32:errorcluster, "JSON Out"=w33:string)  [unwired: 1 in]
      n35 = Greater?(x=w42, y=w23) -> (0:w29:bool)
      n36 = Select(t=1 ("y"), s=w30, f=w39) -> (s? t:f=w31:i32)
      n37 = call "send_command.vi"("error in"=w32, "JSON Command"=w33, "TCP Network Connection in"=w38) -> ("error out"=w44:errorcluster)  [unwired: 1 in, 3 out]
      n38 = Select(t=-1 ("y"), s=w29, f=w31) -> (s? t:f=w41:i32)
    }
    frame "Configure" {
      # "Extract only the information \nwe will be modifying"
      # "Configure initial state for LED and convert configuration to cluster"
      n39 = Unbundle By Name(w98) -> ("Connections.Simulator Connection"=w96:refnum<k5>)
      n40 = call "build_json.vi"("error in"=w99, "Message"=w88, "Command_ID"="VehicleLightsConfig_ID") -> ("error out"=w92:errorcluster, "JSON Out"=w93:string)  [unwired: 1 in]
      n41 = call "send_command.vi"("error in"=w92, "JSON Command"=w93, "TCP Network Connection in"=w96) -> ("error out"=w95:errorcluster)  [unwired: 1 in, 3 out]
      n42 = Unflatten From JSON(JSON string=w88, type and defaults=T10 {"actor_id"="", "lights"=[]} ("Update Config"), error in (no error)=w95) -> (value=w82:T10, error out=w97:errorcluster)  [unwired: 4 in]
      n43 = Unbundle By Name(w82) -> ("actor_id"=w84:string, "lights"=w86:T15)
      n44 = for {
        tunnel: w86 -> [w105] mode=indexing
        tunnel: [w100] -> w83 mode=indexing
        n45 = Unbundle By Name(w105) -> ("array_id"=w102:string, "coneLights"=w104:T16)
        n46 = for {
          tunnel: w104 -> [w110] mode=indexing
          tunnel: [w106] -> w103 mode=indexing
          n47 = Unbundle By Name(w110) -> ("backlight_intensity"=w109:sgl, "intensity"=w108:sgl, "led"=w107:i32)
          n48 = Bundle("backlight_intensity"=w109, "intensity"=w108, "led"=w107) -> (w106:T14)  [unwired: 1 in]
        }
        n49 = Bundle By Name(cluster=T11 {"array_id"="", "coneLights"=[]}, "array_id"=w102, "coneLights"=w103) -> (w100:T11)
      }
      n50 = Bundle By Name(cluster=T9 {"actor_id"="", "lights"=[]} ("Update Intensity"), "actor_id"=w84, "lights"=w83) -> (w81:T9)
    }
    frame "Init", Default {
      # "On replay we need to wait for the car to be spawn before configure lights"
    }
  }
  "error out" <- w18
  n51 = feedback-in #1(w11) -> ()
  n52 = feedback-in #2(w3) -> ()
  n53 = feedback-in #3(w8) -> ()
  n54 = feedback-in #4(w9) -> ()
